vi "Merge Image Manager.vi"(7 "Calling VI Ref":refnum<vi>) -> ()   [LabVIEW 2016]
uses:
  Merge Image Type Defs/Merge Image - Image Control.ctl
  <vilib>/Utility/miscctls.llb/LVPointTypeDef.ctl
  <vilib>/vision/Image Controls.llb/IMAQ Image.ctl
  Merge Image Type Defs/Merge Image - Notifier Type.ctl
  Merge Image Type Defs/Merge Image - Actions.ctl
  <vilib>/vision/NI_Vision_Development_Module.lvlib
panel:
  in  "Blue LUT":cluster{"Blue Min (%)":i32, "Blue Max (%)":i32}={"Blue Min (%)"=0, "Blue Max (%)"=100} {"Blue Max (%)" max=100; "Blue Min (%)" max=100}
  in  "Green LUT":T1={"Green Min (%)"=0, "Green Max (%)"=100} {"Green Max (%)" max=100; "Green Min (%)" max=100}
  in  "Red LUT":cluster{"Red Min (%)":i32, "Red Max (%)":i32}={"Red Min (%)"=0, "Red Max (%)"=100} {"Red Max (%)" max=100; "Red Min (%)" max=100}
  in  "Update Time (ms)":i32=50 min=10 max=300000 step=1
  in  "Load Trans":bool
  in  "Save Trans":bool
  in  "Blue Image":T2 {"Image" items=["None", "Img 01", "Img 02", "Img 03"]}
  in  "Green Image":T2 {"Image" items=["None", "Img 01", "Img 02", "Img 03"]}
  in  "Red Image":T2 {"Image" items=["None", "Img 01", "Img 02", "Img 03"]}
  in  "Image Display":bool
  in  "Quit":bool
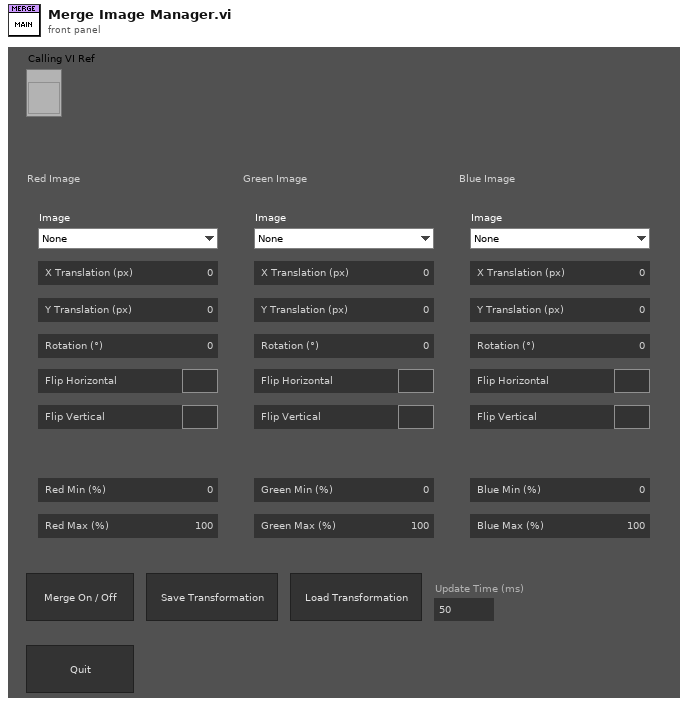
[diagram p1: front panel]
types:
  T1 = cluster{"Green Min (%)":i32, "Green Max (%)":i32}
  T2 = typedef "Merge Image - Image Control.ctl" = cluster{"Image":i32, "X Translation (px)":i32, "Y Translation (px)":i32, "Rotation (°)":sgl, "Flip Horizontal":bool, "Flip Vertical":bool}
  T3 = typedef "Image Type" = u32
  T4 = typedef "Merge Image - Actions.ctl" = enum16{"Timeout", "Update Image Source", "Update LUTs", "Quit"}
  T5 = typedef "Merge Image - Notifier Type.ctl" = cluster{"Actions":T4, "Merge Contols":T2[], "LUT Controls":cluster{"Red Min (%)":i32, "Red Max (%)":i32}[]}
  T6 = typedef "IMAQ Image.ctl" = refnum<image>
  T7 = enum16{"Always On", "Always Off", "Off While Running"}
  T8 = typedef "LVPointTypeDef.ctl" = cluster{"Horizontal":i16, "Vertical":i16}
  T9 = enum32{"Invalid", "Standard", "Closed", "Hidden", "Minimized", "Maximized"}
  T10 = typedef "LVRectTypeDef.ctl" = cluster{"Left":i16, "Top":i16, "Right":i16, "Bottom":i16}
  T11 = typedef "LVBoundsTypeDef.ctl" = cluster{"Width":u32, "Height":u32}
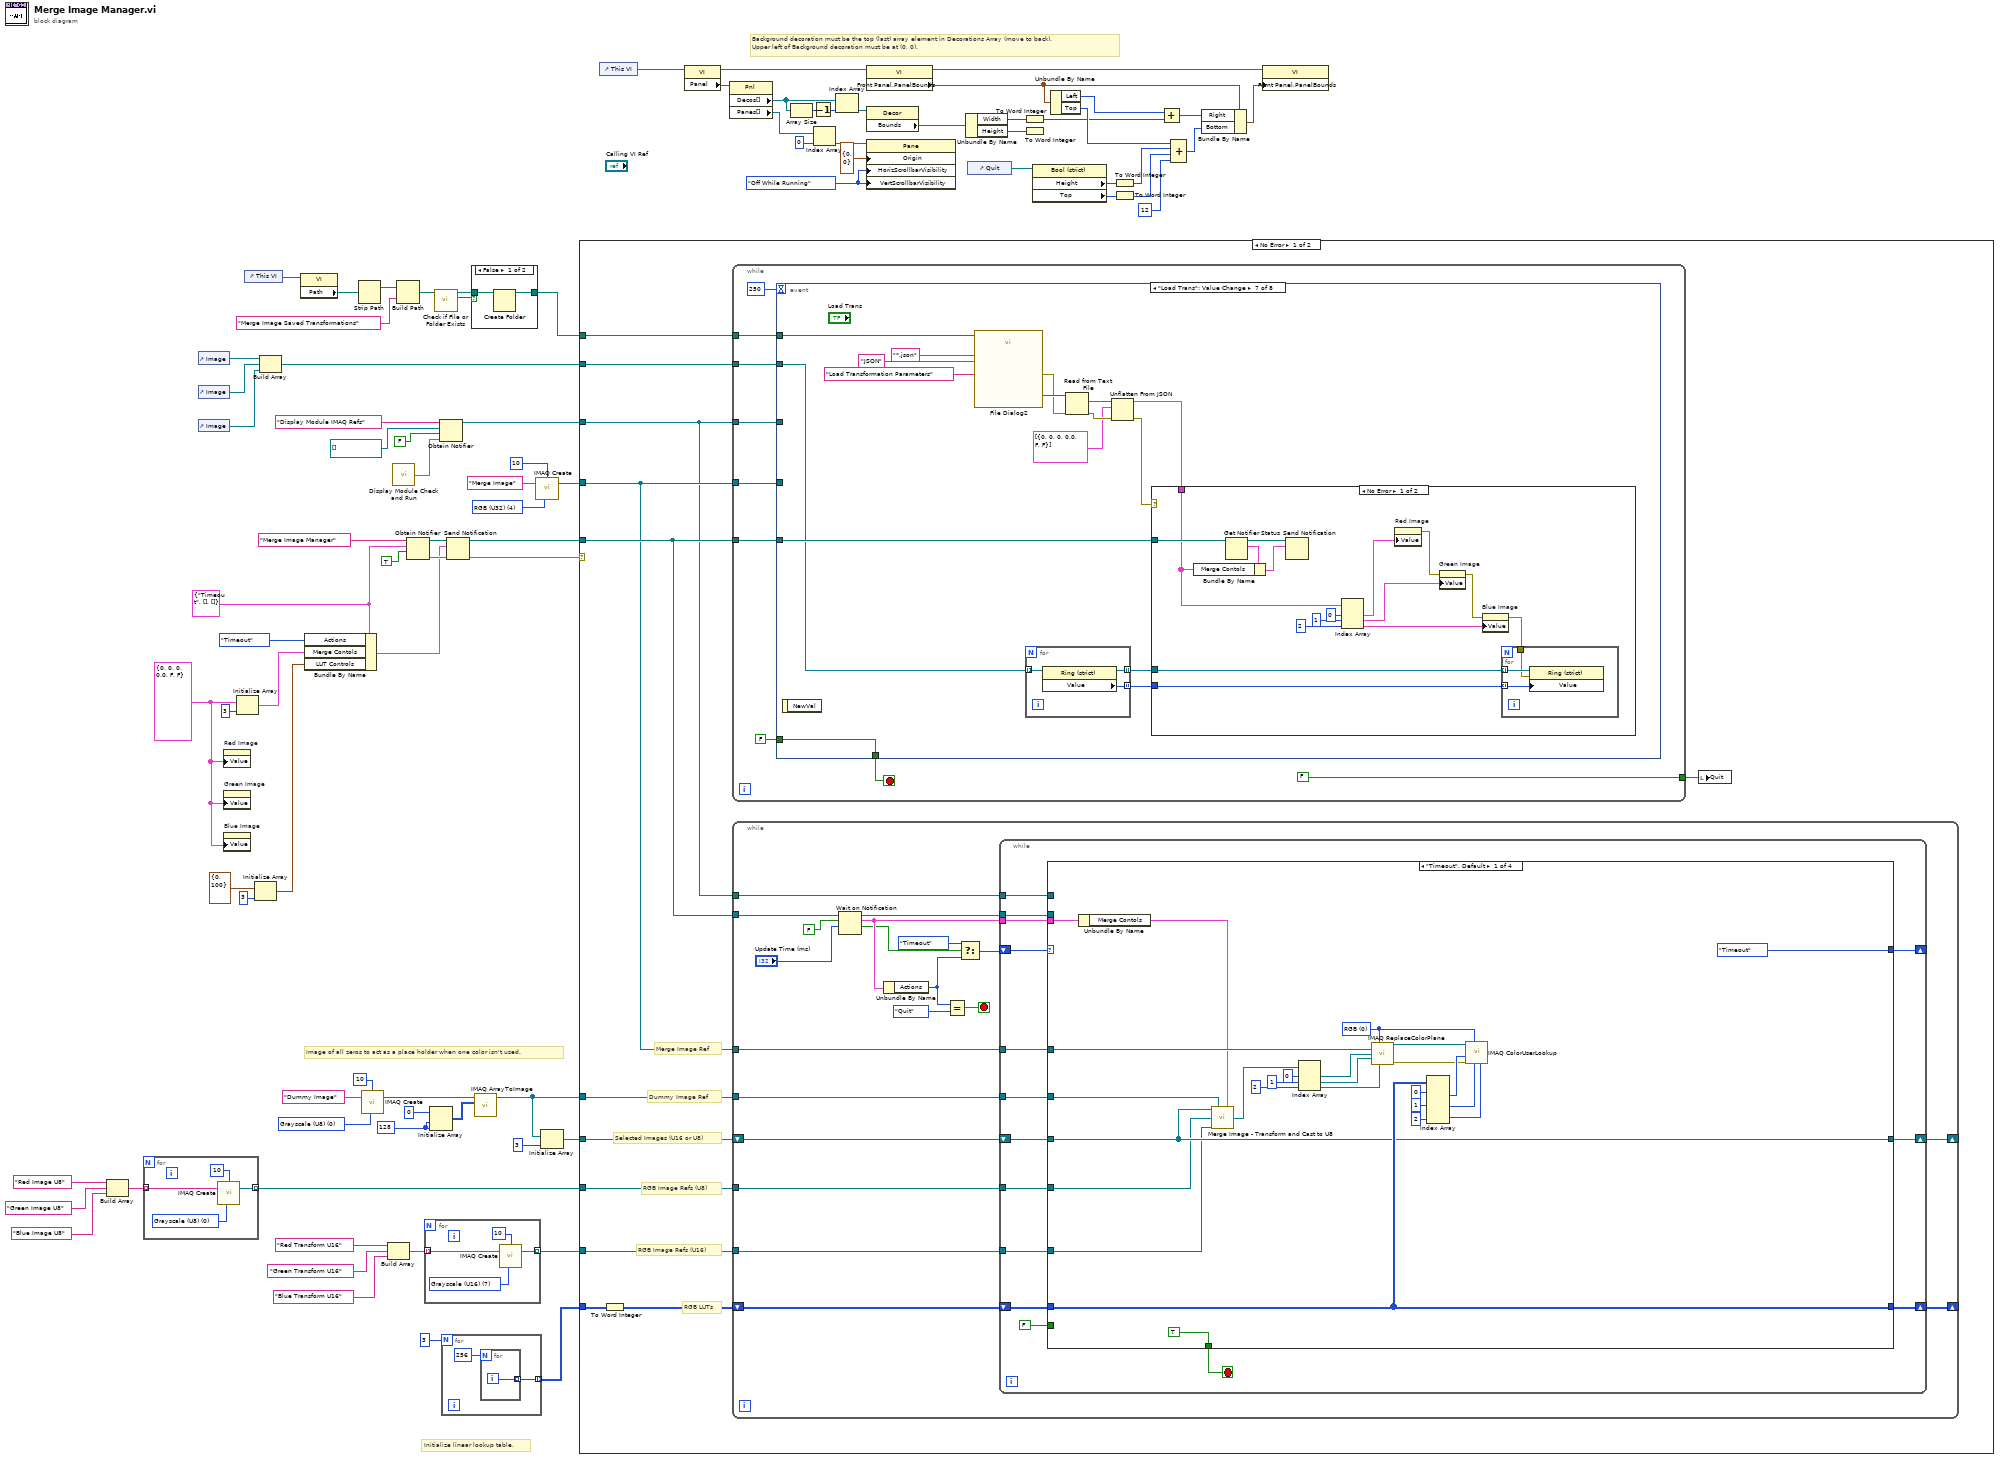
[diagram p0: block diagram]
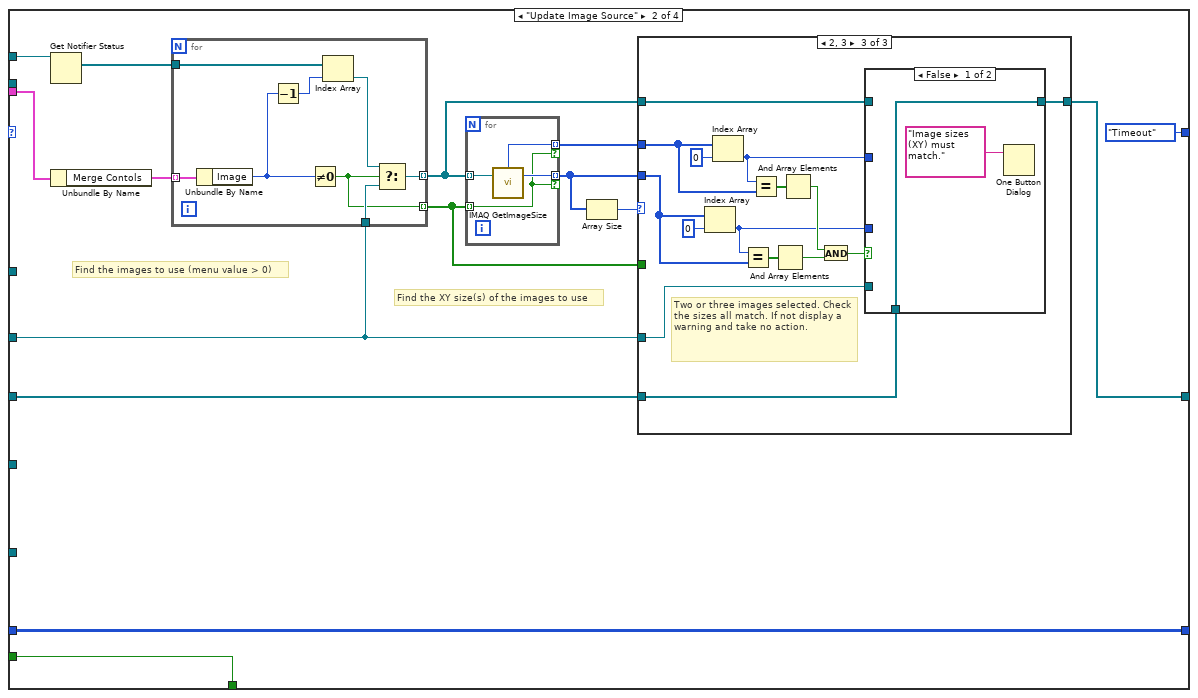
[diagram p3: hidden frame]
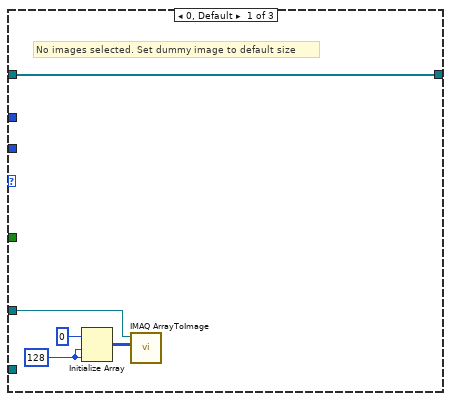
[diagram p4: hidden frame]
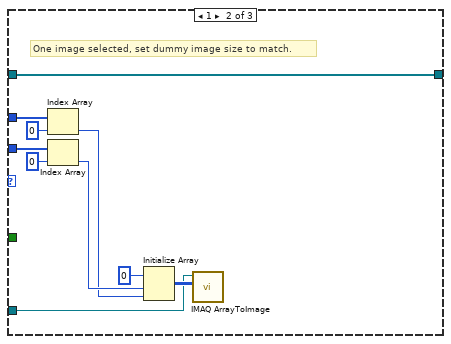
[diagram p5: hidden frame]
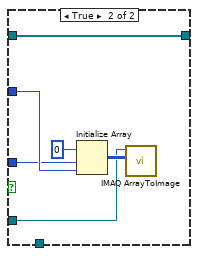
[diagram p6: hidden frame]
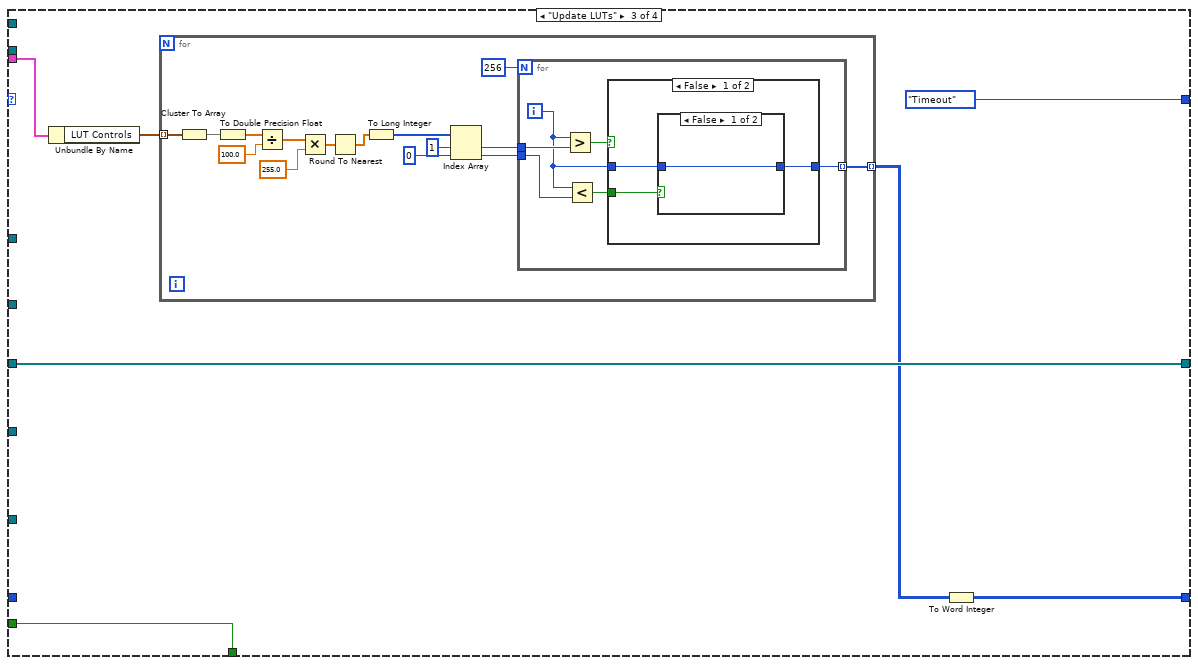
[diagram p7: hidden frame]
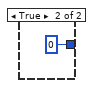
[diagram p8: hidden frame]
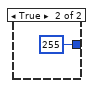
[diagram p9: hidden frame]
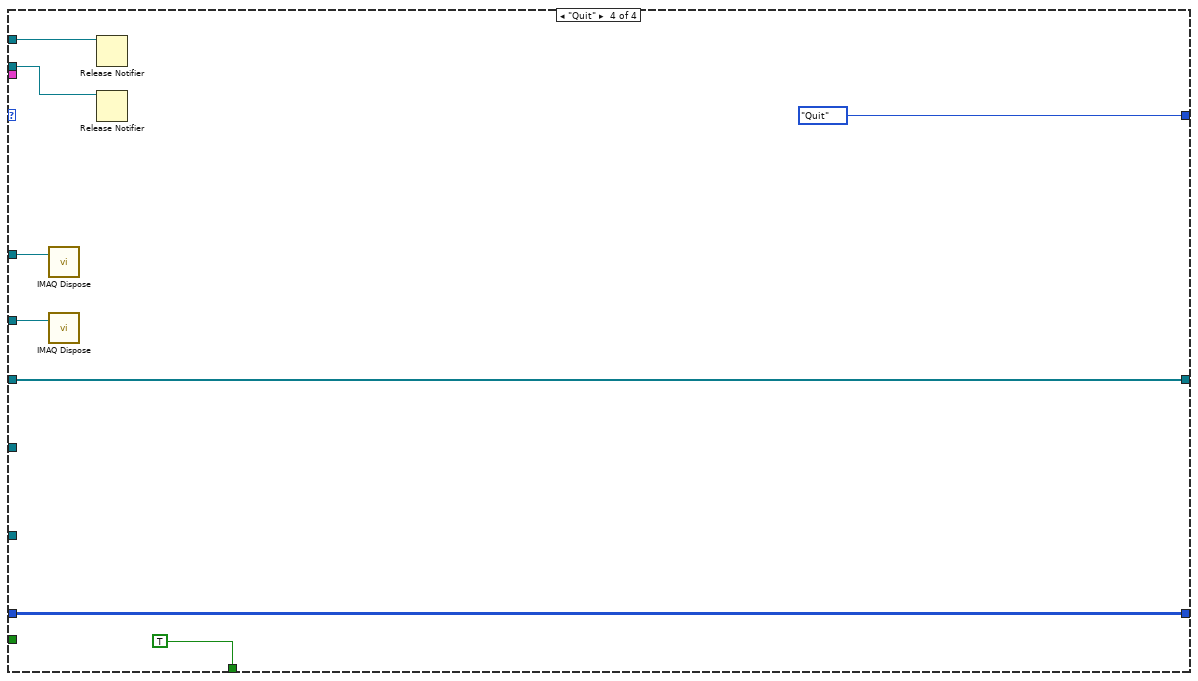
[diagram p10: hidden frame]
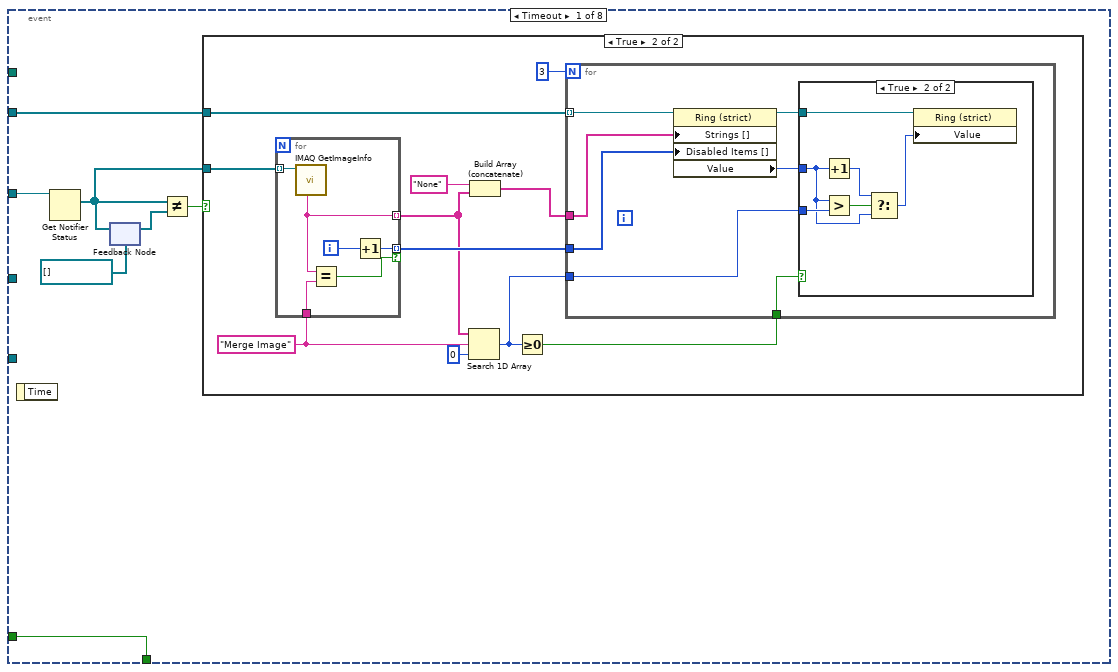
[diagram p11: hidden frame]
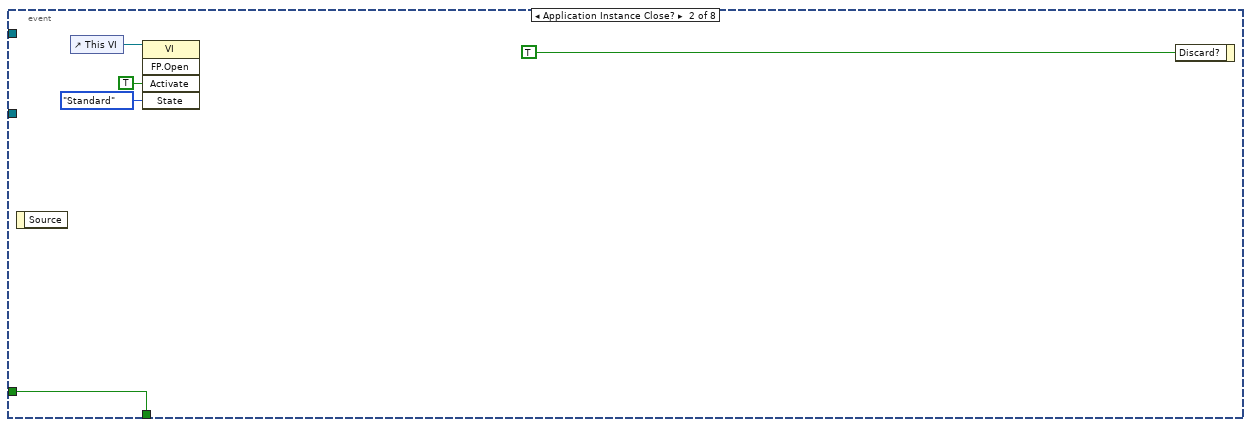
[diagram p14: hidden frame]
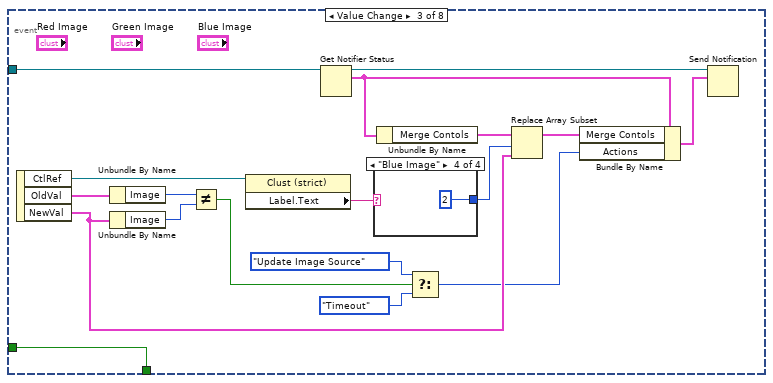
[diagram p15: hidden frame]
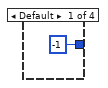
[diagram p16: hidden frame]
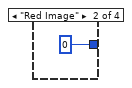
[diagram p17: hidden frame]
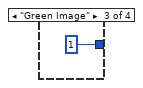
[diagram p18: hidden frame]
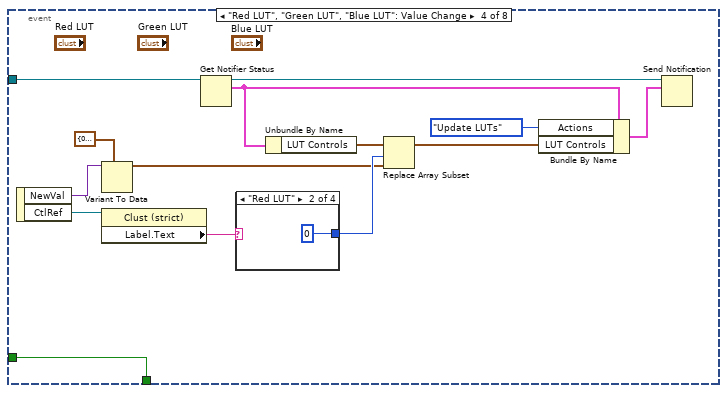
[diagram p19: hidden frame]
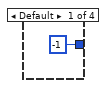
[diagram p20: hidden frame]
diagram:
  w18 = 128 ("dimension size")
  w23 = T3 0 items=["Grayscale (U8)", "Grayscale (I16)", "Grayscale (SGL)", "Complex (CSG)", "RGB (U32)", "HSL (U32)", "RGB (U64)", "Grayscale (U16)"] ("Image Type")
  w2 = T2 {"Image"=0, "X Translation (px)"=0, "Y Translation (px)"=0, "Rotation (°)"=0.0, "Flip Horizontal"=FALSE, "Flip Vertical"=FALSE} ("Image Controls")
  w32 = T5 {"Actions"=enum."Timeout", "Merge Contols"=[], "LUT Controls"=[]} ("Merge Image Notifier Type")
  w41 = T3 4 items=["Grayscale (U8)", "Grayscale (I16)", "Grayscale (SGL)", "Complex (CSG)", "RGB (U32)", "HSL (U32)", "RGB (U64)", "Grayscale (U16)"] ("Image Type")
  w70 = T7."Off While Running" ("Vertical Scrollbar Visibility")
  # "Image of all zeros to act as a place holder when one color isn't used."
  # "Initialize linear lookup table."
  # "Background decoration must be the top (last) array element in Decorations Array (move to back).\nUpper left of Background decoration must be at (0, 0)."
  n1 = Build Array("Red Image U8" ("Image Name"), "Green Image U8" ("Image Name"), "Blue Image U8" ("Image Name")) -> (w12:string[])
  n2 = for {
    tunnel: w12 -> [w89] mode=indexing
    tunnel: [w88] -> w11 mode=indexing
    w90 = T3 0 items=["Grayscale (U8)", "Grayscale (I16)", "Grayscale (SGL)", "Complex (CSG)", "RGB (U32)", "HSL (U32)", "RGB (U64)", "Grayscale (U16)"] ("Image Type")
    n3 = call "IMAQ Create"("Border Size"=10, "Image Name"=w89, "Image Type"=w90) -> ("New Image"=w88:T6)  [unwired: 2 in, 1 out]
  }
  n4 = control-ref of="Image"() -> (w37:refnum<vi>)
  n5 = control-ref of="Image"() -> (w35:refnum<vi>)
  n6 = control-ref of="Image"() -> (w36:refnum<vi>)
  n7 = property on="Red Image" class="Clust (strict)"("Value"=w2) -> ()  [unwired: 2 in, 2 out]
  n8 = property on="Green Image" class="Clust (strict)"("Value"=w2) -> ()  [unwired: 2 in, 2 out]
  n9 = property on="Blue Image" class="Clust (strict)"("Value"=w2) -> ()  [unwired: 2 in, 2 out]
  n10 = Initialize Array(w2, 3 ("dimension size")) -> (w29:T2[])
  n11 = control-ref of="This VI"() -> (w54:refnum<vi>)
  n12 = Initialize Array(cluster{"Red Min (%)":i32, "Red Max (%)":i32} {"Red Min (%)"=0, "Red Max (%)"=100} ("LUT Controls"), 3 ("dimension size")) -> (w26:cluster{"Red Min (%)":i32, "Red Max (%)":i32}[])
  n13 = Build Array(w37, w35, w36) -> (w34:refnum<vi>[])
  n14 = property class="VI"(reference=w54) -> ("Path"=w53:path)  [unwired: 1 in, 2 out]
  n15 = Bundle By Name(cluster=w32, "Actions"=Merge_Image_-_Actions."Timeout", "Merge Contols"=w29, "LUT Controls"=w26) -> (w25:T5)
  n16 = Strip Path(path=w53) -> (stripped path=w52:path)  [unwired: 1 out]
  n17 = call "IMAQ Create"("Border Size"=10, "Image Name"="Dummy Image", "Image Type"=w23) -> ("New Image"=w24:T6)  [unwired: 2 in, 1 out]
  n18 = Build Array("Red Transform U16" ("Image Name"), "Green Transform U16" ("Image Name"), "Blue Transform U16" ("Image Name")) -> (w7:string[])
  n19 = call "Display Module Check and Run.vi"() -> ("Error"=w33:errorcluster)  [unwired: 15 in]
  n20 = Build Path(base path=w52, name or relative path="Merge Image Saved Transformations") -> (appended path=w50:path)
  n21 = Obtain Notifier(name (unnamed)="Merge Image Manager", notification data type=w32, create if not found? (T)=TRUE) -> (notifier out=w56:refnum<notifier>, error out=w47:errorcluster)  [unwired: 1 in, 1 out]
  n22 = for {
    tunnel: w7 -> [w93] mode=indexing
    tunnel: [w92] -> w3 mode=indexing
    w94 = T3 7 items=["Grayscale (U8)", "Grayscale (I16)", "Grayscale (SGL)", "Complex (CSG)", "RGB (U32)", "HSL (U32)", "RGB (U64)", "Grayscale (U16)"] ("Image Type")
    n23 = call "IMAQ Create"("Border Size"=10, "Image Name"=w93, "Image Type"=w94) -> ("New Image"=w92:T6)  [unwired: 2 in, 1 out]
  }
  n24 = Initialize Array(u8 0 ("element"), w18, w18) -> (w19:u8[][])
  n25 = call <vilib>:"Check if File or Folder Exists.vi"("path"=w50) -> ("file or folder exists?"=w49:bool, "dup path"=w48:path)  [unwired: 8 in, 1 out]
  n26 = Obtain Notifier(name (unnamed)="Display Module IMAQ Refs", notification data type=T6[] [], create if not found? (T)=FALSE, error in (no error)=w33) -> (notifier out=w38:refnum<notifier>)  [unwired: 2 out]
  n27 = for {
    N: 3 -> [_]
    tunnel: [w96] -> w16 mode=indexing
    n28 = for {
      N: 256 -> [_]
      tunnel: [w98] -> w96 mode=indexing
      i -> [w98]
    }
  }
  n29 = Send Notification(notification=w25, notifier=w56, error in (no error)=w47) -> (notifier out=w55:refnum<notifier>, error out=w46:errorcluster)
  n30 = case shown="False" w49 {
    tunnel: w48 -> [w100 w101]
    tunnel: [w99 w101] -> w1
    frame False {
      n31 = Create Folder(path (use dialog)=w100) -> (created path=w99:path)  [unwired: 2 in, 2 out]
    }
    frame True {
    }
  }
  n32 = call "IMAQ ArrayToImage"("Image Pixels (U8)"=w19, "Image"=w24) -> ("Image Out"=w8:T6)  [unwired: 8 in, 1 out]
  n33 = call "IMAQ Create"("Border Size"=10, "Image Name"="Merge Image", "Image Type"=w41) -> ("New Image"=w39:T6)  [unwired: 2 in, 1 out]
  n34 = Initialize Array(w8, 3 ("dimension size")) -> (w9:T6[])
  n35 = case shown="No Error" w46 {
    selector: w46 -> [_ w471]
    tunnel: w55 -> [w112 w473]
    tunnel: w39 -> [w108 w472]
    tunnel: w38 -> [w107 w474]
    tunnel: w34 -> [w111 _]
    tunnel: w8 -> [w110 _]
    tunnel: w11 -> [w106 _]
    tunnel: w16 -> [w109 _]
    tunnel: w9 -> [w105 _]
    tunnel: w3 -> [w104 _]
    tunnel: w1 -> [w102 _]
    frame No Error {
      # "RGB Image Refs (U16)"
      # "Selected Images (U16 or U8)"
      # "Merge Image Ref"
      # "Dummy Image Ref"
      # "RGB Image Refs (U8)"
      # "RGB LUTs"
      n36 = To Word Integer(number=w109) -> (16bit integer=w103:i16[][])
      n37 = while {
        tunnel: w112 -> [w288]
        tunnel: [FALSE] -> w113
        tunnel: w108 -> [w286]
        tunnel: w107 -> [w285]
        tunnel: w111 -> [w284]
        tunnel: w102 -> [w282]
        stop <- w289 stop-if-true
        n38 = event shown="[6] \"Load Trans\": Value Change" {
          selector: _ -> [_ _ _ _ _ _ _ _]
          dyn-events: _ -> [_ _ _ _ _ _ _ _]
          timeout: 250 -> [_ _ _ _ _ _ _ _]
          tunnel: FALSE -> [w297 w331 w350 w368 w383 w422 w440 _]
          tunnel: [w297 w331 w350 w368 w383 w422 w440 w468] -> w289
          tunnel: w288 -> [_ _ w349 w367 _ w421 w430 w467]
          tunnel: w286 -> [_ _ _ _ w375 _ _ _]
          tunnel: w285 -> [w296 _ _ _ w374 _ _ _]
          tunnel: w284 -> [w292 _ _ _ w373 _ w427 _]
          tunnel: w282 -> [_ _ _ _ _ w418 w435 _]
          event Timeout {
            n39 = event-data() -> ()  [unwired: 1 in, 1 out]
            n40 = Get Notifier Status(notifier=w296) -> (current notification=w291:T6[])  [unwired: 1 in, 4 out]
            n41 = feedback-in #1(w291) -> ()
            n42 = feedback #1(T6[] []) -> (w294:T6[])
            n43 = Not Equal?(x=w291, y=w294) -> (x != y?=w293:bool)
            n44 = case shown="True" w293 {
              tunnel: w292 -> [_ w307]
              tunnel: w291 -> [_ w308]
              frame False {
              }
              frame True {
                w301 = "Merge Image" ("Image Name")
                n45 = for {
                  tunnel: w308 -> [w327] mode=indexing
                  tunnel: [w326] -> w302 mode=indexing
                  tunnel: [w325] -> w303 mode=indexing if=w323
                  tunnel: w301 -> [w322]
                  i -> [w324]
                  n46 = call "IMAQ GetImageInfo"("Image"=w327) -> ("Image Name"=w326:string)  [unwired: 3 in, 7 out]
                  n47 = Equal?(x=w326, y=w322) -> (x = y?=w323:bool)
                  n48 = Increment(x=w324) -> (x+1=w325:i32)
                }
                n49 = Search 1D Array(1D array=w302, element=w301, start index (0)=0) -> (index of element=w298:i32)
                n50 = Build Array (concatenate)("None", w302) -> (w305:string[])
                n51 = Greater Or Equal To 0?(x=w298) -> (x >= 0?=w299:bool)
                n52 = for {
                  N: 3 -> [_]
                  tunnel: w307 -> [w315] mode=indexing
                  tunnel: w305 -> [w314]
                  tunnel: w303 -> [w313]
                  tunnel: w299 -> [w310]
                  tunnel: w298 -> [w309]
                  n53 = property class="Ring (strict)"(reference=w315, "Strings []"=w314, "Disabled Items []"=w313) -> (reference out=w312:refnum<vi>, "Value"=w311:i32)  [unwired: 1 in, 1 out]
                  n54 = case shown="True" w310 {
                    tunnel: w312 -> [_ w321]
                    tunnel: w311 -> [_ w316]
                    tunnel: w309 -> [_ w320]
                    frame False {
                    }
                    frame True {
                      n55 = Increment(x=w316) -> (x+1=w318:i32)
                      n56 = Greater?(x=w316, y=w320) -> (0:w319:bool)
                      n57 = Select(t=w318, s=w319, f=w316) -> (s? t:f=w317:i32)
                      n58 = property class="Ring (strict)"(reference=w321, "Value"=w317) -> ()  [unwired: 1 in, 2 out]
                    }
                  }
                }
              }
            }
          }
          event Application Instance Close? {
            n59 = event-data() -> ()  [unwired: 1 in, 1 out]
            n60 = control-ref of="This VI"() -> (w328:refnum<vi>)
            n61 = invoke class="VI" method="FP.Open"(reference=w328, "Activate"=TRUE ("Activate?"), "State"=T9."Standard") -> ()  [unwired: 2 in, 5 out]
            n62 = event-data("Discard?"=TRUE) -> ()  [unwired: 1 in, 1 out]
          }
          event Value Change {
            n63 = event-data() -> ("CtlRef"=w347:refnum<vi>, "OldVal"=w340:T2, "NewVal"=w337:T2)  [unwired: 1 in]
            n64 = Unbundle By Name(w340) -> ("Image"=w339:i32)
            n65 = Unbundle By Name(w337) -> ("Image"=w338:i32)
            n66 = Not Equal?(x=w339, y=w338) -> (x != y?=w336:bool)
            n67 = property class="Clust (strict)"(reference=w347) -> ("Label.Text"=w346:string)  [unwired: 1 in, 2 out]
            n68 = Get Notifier Status(notifier=w349) -> (notifier out=w348:refnum<notifier>, current notification=w341:T5)  [unwired: 1 in, 3 out]
            n69 = case shown="\"Blue Image\"" w346 {
              tunnel: [-1 0 1 2] -> w344
              frame Default {
              }
              frame "Red Image" {
              }
              frame "Green Image" {
              }
              frame "Blue Image" {
              }
            }
            n70 = Unbundle By Name(w341) -> ("Merge Contols"=w345:T2[])
            n71 = Select(t=Merge_Image_-_Actions."Update Image Source" ("Actions"), s=w336, f=Merge_Image_-_Actions."Timeout" ("Actions")) -> (s? t:f=w333:T4)
            n72 = Replace Array Subset(array=w345, new element=w337, index=w344) -> (w343:T2[])
            n73 = Bundle By Name(cluster=w341, "Merge Contols"=w343, "Actions"=w333) -> (w342:T5)
            n74 = Send Notification(notification=w342, notifier=w348) -> ()  [unwired: 1 in, 2 out]
          }
          event "Red LUT", "Green LUT", "Blue LUT": Value Change {
            n75 = event-data() -> ("NewVal"=w357:variant, "CtlRef"=w358:refnum<vi>)  [unwired: 1 in]
            n76 = Variant To Data(type=cluster{"Red Min (%)":u16, "Red Max (%)":u16} {"Red Min (%)"=0, "Red Max (%)"=100} ("LUT Controls"), Variant=w357) -> (data=w355:cluster{"Red Min (%)":u16, "Red Max (%)":u16})  [unwired: 1 in, 1 out]
            n77 = property class="Clust (strict)"(reference=w358) -> ("Label.Text"=w365:string)  [unwired: 1 in, 2 out]
            n78 = Get Notifier Status(notifier=w367) -> (notifier out=w366:refnum<notifier>, current notification=w359:T5)  [unwired: 1 in, 3 out]
            n79 = case shown="\"Red LUT\"" w365 {
              tunnel: [-1 0 1 2] -> w363
              frame Default {
              }
              frame "Red LUT" {
              }
              frame "Green LUT" {
              }
              frame "Blue LUT" {
              }
            }
            n80 = Unbundle By Name(w359) -> ("LUT Controls"=w364:cluster{"Red Min (%)":i32, "Red Max (%)":i32}[])
            n81 = Replace Array Subset(array=w364, new element=w355, index=w363) -> (w362:cluster{"Red Min (%)":i32, "Red Max (%)":i32}[])
            n82 = Bundle By Name(cluster=w359, "Actions"=Merge_Image_-_Actions."Update LUTs", "LUT Controls"=w362) -> (w360:T5)
            n83 = Send Notification(notification=w360, notifier=w366) -> ()  [unwired: 1 in, 2 out]
          }
          event "Image Display": Value Change {
            n84 = event-data() -> ("NewVal"=w376:bool)  [unwired: 1 in]
            n85 = Get Notifier Status(notifier=w374) -> (notifier out=w382:refnum<notifier>, current notification=w380:T6[], error out=w381:errorcluster)  [unwired: 1 in, 2 out]
            n86 = case shown="False" w376 {
              tunnel: w382 -> [w392 w409]
              tunnel: w381 -> [w390 w408]
              tunnel: w380 -> [w389 w407]
              tunnel: [w391 w405] -> w377
              tunnel: [w392 w409] -> w379
              tunnel: [w390 w408] -> w378
              tunnel: w375 -> [w388 w406]
              tunnel: w373 -> [w385 _]
              frame False {
                n87 = Search 1D Array(1D array=w389, element=w388, start index (0)=0) -> (index of element=w384:i32)
                n88 = Greater Or Equal To 0?(x=w384) -> (x >= 0?=w386:bool)
                n89 = case shown="True" w386 {
                  tunnel: w384 -> [_ w403]
                  tunnel: w389 -> [w400 w402]
                  tunnel: [w400 w401] -> w391
                  frame False {
                  }
                  frame True {
                    n90 = Delete From Array(array=w402, length=1, index=w403) -> (array with subset deleted=w401:T6[])  [unwired: 1 out]
                  }
                }
                n91 = for {
                  tunnel: w385 -> [w399] mode=indexing
                  tunnel: w384 -> [w397]
                  n92 = property class="Ring (strict)"(reference=w399) -> (reference out=w398:refnum<vi>, "Value"=w393:i32)  [unwired: 1 in, 1 out]
                  n93 = Greater?(x=w393, y=w397) -> (0:w396:bool)
                  n94 = Decrement(x=w393) -> (x-1=w395:i32)
                  n95 = Select(t=w395, s=w396, f=w393) -> (s? t:f=w394:i32)
                  n96 = property class="Ring (strict)"(reference=w398, "Value"=w394) -> ()  [unwired: 1 in, 2 out]
                }
              }
              frame True {
                n97 = Build Array (concatenate)(w407, w406) -> (w405:T6[])
              }
            }
            n98 = Send Notification(notification=w377, notifier=w379, error in (no error)=w378) -> ()  [unwired: 2 out]
          }
          event "Save Trans": Value Change {
            n99 = event-data() -> ()  [unwired: 1 in, 1 out]
            n100 = Get Notifier Status(notifier=w421) -> (current notification=w420:T5, error out=w411:errorcluster)  [unwired: 1 in, 3 out]
            n101 = Unbundle By Name(w420) -> ("Merge Contols"=w419:T2[])
            n102 = Flatten To JSON(anything=w419, error in (no error)=w411) -> (JSON string=w412:string, 11:w410:errorcluster)  [unwired: 1 in]
            n103 = call "File Dialog"("start path"=w418, "prompt"="Save Transformation Parameters", "error in"=w410, "pattern (all files)"="*.json", "pattern label"="JSON") -> ("selected path"=w413:path, "error out"=w414:errorcluster)  [unwired: 7 in, 2 out]
            n104 = case shown="No Error" w414 {
              tunnel: w413 -> [w424 _]
              tunnel: w412 -> [w423 _]
              frame No Error {
                n105 = Write to Text File(file (use dialog)=w424, text=w423) -> ()  [unwired: 2 in, 3 out]
              }
              frame Error {
              }
            }
          }
          event "Load Trans": Value Change {
            n106 = event-data() -> ()  [unwired: 1 in, 1 out]
            n107 = call "File Dialog2"("start path"=w435, "prompt"="Load Transformation Parameters", "pattern (all files)"="*.json", "pattern label"="JSON") -> ("selected path"=w436:path, "error out"=w434:errorcluster)  [unwired: 8 in, 2 out]
            n108 = for {
              tunnel: w427 -> [w443] mode=indexing
              tunnel: [w442] -> w425 mode=indexing
              tunnel: [w441] -> w426 mode=indexing
              n109 = property class="Ring (strict)"(reference=w443) -> (reference out=w441:refnum<vi>, "Value"=w442:i32)  [unwired: 1 in, 1 out]
            }
            n110 = Read from Text File(file (use dialog)=w436, error in=w434) -> (text=w433:string, error out=w432:errorcluster)  [unwired: 2 in, 2 out]
            n111 = Unflatten From JSON(JSON string=w433, type and defaults=T2[] [{"Image"=0, "X Translation (px)"=0, "Y Translation (px)"=0, "Rotation (°)"=0.0, "Flip Horizontal"=FALSE, "Flip Vertical"=FALSE}], error in (no error)=w432) -> (value=w429:T2[], error out=w428:errorcluster)  [unwired: 4 in]
            n112 = case shown="No Error" w428 {
              tunnel: w430 -> [w459 _]
              tunnel: w429 -> [w455 _]
              tunnel: w426 -> [w448 _]
              tunnel: w425 -> [w447 _]
              frame No Error {
                n113 = Get Notifier Status(notifier=w459) -> (notifier out=w458:refnum<notifier>, current notification=w457:T5)  [unwired: 1 in, 3 out]
                n114 = Bundle By Name(cluster=w457, "Merge Contols"=w455) -> (w456:T5)
                n115 = Send Notification(notification=w456, notifier=w458) -> ()  [unwired: 1 in, 2 out]
                n116 = Index Array(array=w455, index #1=0 ("index"), index #2=1 ("index"), index #3=2 ("index")) -> (element #1=w451:T2, element #2=w450:T2, element #3=w449:T2)
                n117 = property on="Red Image" class="Clust (strict)"("Value"=w451) -> (error out=w446:errorcluster)  [unwired: 2 in, 1 out]
                n118 = property on="Green Image" class="Clust (strict)"(error in=w446, "Value"=w450) -> (error out=w445:errorcluster)  [unwired: 1 in, 1 out]
                n119 = property on="Blue Image" class="Clust (strict)"(error in=w445, "Value"=w449) -> (error out=w444:errorcluster)  [unwired: 1 in, 1 out]
                n120 = for {
                  tunnel: w448 -> [w462] mode=indexing
                  tunnel: w447 -> [w461] mode=indexing
                  tunnel: w444 -> [w460]
                  n121 = property class="Ring (strict)"(reference=w462, error in=w460, "Value"=w461) -> ()  [unwired: 2 out]
                }
              }
              frame Error {
              }
            }
          }
          event "Quit": Value Change {
            n122 = event-data() -> ("NewVal"=w468:bool)  [unwired: 1 in]
            n123 = Get Notifier Status(notifier=w467) -> (notifier out=w466:refnum<notifier>, current notification=w465:T5)  [unwired: 1 in, 3 out]
            n124 = Bundle By Name(cluster=w465, "Actions"=Merge_Image_-_Actions."Quit") -> (w463:T5)
            n125 = Send Notification(notification=w463, notifier=w466) -> ()  [unwired: 1 in, 2 out]
          }
        }
      }
      n126 = while {
        tunnel: w112 -> [w133]
        tunnel: w110 -> [w122]
        shift-right: [w119] -> _
        shift-left: w105 -> [w121]
        shift-right: [w118] -> _
        shift-left: w103 -> [w120]
        tunnel: w108 -> [w117]
        tunnel: w107 -> [w116]
        tunnel: w106 -> [w115]
        tunnel: w104 -> [w114]
        stop <- w131 stop-if-true
        n127 = Wait on Notification(notifier=w133, ignore previous (F)=FALSE, timeout in ms (-1)="Update Time (ms)") -> (notifier out=w129:refnum<notifier>, notification=w130:T5, timed out?=w127:bool)  [unwired: 1 in, 1 out]
        n128 = Unbundle By Name(w130) -> ("Actions"=w126:T4)
        n129 = Equal?(x=w126, y=Merge_Image_-_Actions."Quit") -> (x = y?=w131:bool)
        n130 = Select(t=Merge_Image_-_Actions."Timeout", s=w127, f=w126) -> (s? t:f=w124:T4)
        n131 = while {
          shift-right: [w146] -> _
          shift-left: w124 -> [w148]
          tunnel: w130 -> [w147]
          tunnel: w129 -> [w145]
          tunnel: w122 -> [w142]
          tunnel: w117 -> [w136]
          tunnel: w116 -> [w137]
          shift-right: [w139] -> w119
          shift-left: w121 -> [w141]
          tunnel: w115 -> [w135]
          tunnel: w114 -> [w134]
          shift-right: [w138] -> w118
          shift-left: w120 -> [w140]
          stop <- w143 stop-if-true
          n132 = case shown="\"Timeout\", Default" w148 {
            tunnel: w147 -> [w168 w186 w243 _]
            tunnel: [Merge_Image_-_Actions."Timeout" ("y") Merge_Image_-_Actions."Timeout" ("y") Merge_Image_-_Actions."Timeout" ("y") Merge_Image_-_Actions."Quit" ("y")] -> w146
            tunnel: w145 -> [_ _ _ w275]
            tunnel: FALSE -> [_ w189 w245 _]
            tunnel: [TRUE w189 w245 TRUE] -> w143
            tunnel: w142 -> [w167 w175 _ w279]
            tunnel: w141 -> [w171 w176 w244 w277]
            tunnel: w140 -> [w172 w187 _ w278]
            tunnel: [w171 w177 w244 w277] -> w139
            tunnel: [w172 w187 w240 w278] -> w138
            tunnel: w137 -> [_ w184 _ w274]
            tunnel: w136 -> [w173 _ _ w276]
            tunnel: w135 -> [w170 _ _ _]
            tunnel: w134 -> [w169 _ _ _]
            frame "Timeout", Default {
              w157 = u16 0 items=["RGB", "HSL", "HSV", "HSI"] ("Color Mode")
              n133 = Unbundle By Name(w168) -> ("Merge Contols"=w166:T2[])
              n134 = call "Merge Image - Transform and Cast to U8.vi"("Selected Image (U8 or U16)"=w171, "Dummy Image Ref"=w167, "Transform Parameters"=w166, "RGB Image Refs (U8)"=w170, "RGB Image Refs (U16)"=w169) -> ("RGB Image Refs (U8 DUP)"=w165:T6[])  [unwired: 10 in]
              n135 = Index Array(array=w165, index #1=0 ("index"), index #2=1 ("index"), index #3=2 ("index")) -> (element #1=w161:T6, element #2=w160:T6, element #3=w159:T6)
              n136 = call "IMAQ ReplaceColorPlane"("Color Mode"=w157, "Image Dst"=w173, "Red or Hue Plane"=w161, "Green or Sat Plane"=w160, "Blue or Luma or Val or Inten Plane"=w159) -> ("Image Dst Out"=w150:T6, "error out"=w149:errorcluster)  [unwired: 9 in]
              n137 = Index Array(array=w172, index (row) #1=0 ("index (row)"), index (row) #2=1 ("index (row)"), index (row) #3=2 ("index (row)")) -> (element #1=w153:i16[], element #2=w152:i16[], element #3=w151:i16[])  [unwired: 3 in]
              n138 = call "IMAQ ColorUserLookup"("Blue or Luma or Val or Inten Lookup Table"=w151, "Green or Sat Lookup Table"=w152, "Color Mode"=w157, "error in (no error)"=w149, "Red or Hue Lookup Table"=w153, "Image Src"=w150) -> ()  [unwired: 4 in, 2 out]
            }
            frame "Update Image Source" {
              # "Find the XY size(s) of the images to use"
              # "Find the images to use (menu value > 0)"
              n139 = Get Notifier Status(notifier=w184) -> (current notification=w183:T6[])  [unwired: 1 in, 4 out]
              n140 = Unbundle By Name(w186) -> ("Merge Contols"=w185:T2[])
              n141 = for {
                tunnel: w185 -> [w239] mode=indexing
                tunnel: w183 -> [w238]
                tunnel: [w234] -> w178 mode=indexing
                tunnel: w175 -> [w233]
                tunnel: [w232] -> w179 mode=indexing
                n142 = Unbundle By Name(w239) -> ("Image"=w237:i32)
                n143 = Decrement(x=w237) -> (x-1=w236:i32)
                n144 = Not Equal To 0?(x=w237) -> (x != 0?=w232:bool)
                n145 = Index Array(array=w238, index=w236) -> (element=w235:T6)
                n146 = Select(t=w235, s=w232, f=w233) -> (s? t:f=w234:T6)
              }
              n147 = for {
                tunnel: w178 -> [w231] mode=indexing
                tunnel: w179 -> [w228] mode=indexing
                tunnel: [w230] -> w181 mode=indexing if=w228
                tunnel: [w229] -> w180 mode=indexing if=w228
                n148 = call "IMAQ GetImageSize"("Image"=w231) -> ("Y Resolution"=w229:i32, "X Resolution"=w230:i32)  [unwired: 3 in, 1 out]
              }
              n149 = Array Size(array=w180) -> (size(s)=w182:i32)
              n150 = case shown="2, 3" w182 {
                tunnel: w181 -> [_ w204 w214]
                tunnel: w180 -> [_ w201 w217]
                tunnel: w179 -> [_ _ _]
                tunnel: w178 -> [w191 w196 w208]
                tunnel: [w191 w196 w207] -> w177
                tunnel: w176 -> [_ _ w206]
                tunnel: w175 -> [w190 w195 w205]
                frame 0, Default {
                  w193 = 128 ("dimension size")
                  # "No images selected. Set dummy image to default size"
                  n151 = Initialize Array(u8 0 ("element"), w193, w193) -> (w192:u8[][])
                  n152 = call "IMAQ ArrayToImage"("Image Pixels (U8)"=w192, "Image"=w190) -> ()  [unwired: 8 in, 2 out]
                }
                frame 1 {
                  # "One image selected, set dummy image size to match."
                  n153 = Index Array(array=w204, index=0) -> (element=w197:i32)
                  n154 = Index Array(array=w201, index=0) -> (element=w198:i32)
                  n155 = Initialize Array(u8 0 ("element"), w198, w197) -> (w199:u8[][])
                  n156 = call "IMAQ ArrayToImage"("Image Pixels (U8)"=w199, "Image"=w195) -> ()  [unwired: 8 in, 2 out]
                }
                frame 2, 3 {
                  # "Two or three images selected. Check the sizes all match. If not display a warning and take no action."
                  n157 = Index Array(array=w217, index=0) -> (element=w209:i32)
                  n158 = Index Array(array=w214, index=0) -> (element=w210:i32)
                  n159 = Equal?(x=w209, y=w217) -> (x = y?=w216:bool[])
                  n160 = Equal?(x=w210, y=w214) -> (x = y?=w215:bool[])
                  n161 = And Array Elements(Boolean array=w216) -> (logical AND=w212:bool)
                  n162 = And Array Elements(Boolean array=w215) -> (logical AND=w213:bool)
                  n163 = And(x=w213, y=w212) -> (x .and. y?=w211:bool)
                  n164 = case shown="False" w211 {
                    tunnel: w210 -> [_ w224]
                    tunnel: w209 -> [_ w223]
                    tunnel: w208 -> [_ w227]
                    tunnel: [w221 w227] -> w207
                    tunnel: w205 -> [_ w222]
                    tunnel: w206 -> [w221 _]
                    frame False {
                      n165 = One Button Dialog(message="Image sizes (XY) must match.") -> ()  [unwired: 1 in, 1 out]
                    }
                    frame True {
                      n166 = Initialize Array(u8 0 ("element"), w223, w224) -> (w225:u8[][])
                      n167 = call "IMAQ ArrayToImage"("Image Pixels (U8)"=w225, "Image"=w222) -> ()  [unwired: 8 in, 2 out]
                    }
                  }
                }
              }
            }
            frame "Update LUTs" {
              n168 = Unbundle By Name(w243) -> ("LUT Controls"=w242:cluster{"Red Min (%)":i32, "Red Max (%)":i32}[])
              n169 = for {
                tunnel: w242 -> [w261] mode=indexing
                tunnel: [w257] -> w241 mode=indexing
                n170 = Cluster To Array(cluster=w261) -> (array=w256:i32[])
                n171 = To Double Precision Float(number=w256) -> (double precision float=w255:dbl[])
                n172 = Divide(x=w255, y=100.0) -> (x/y=w253:dbl[])
                n173 = Multiply(x=w253, y=255.0) -> (x*y=w251:dbl[])
                n174 = Round To Nearest(number=w251) -> (nearest integer value=w249:dbl[])
                n175 = To Long Integer(number=w249) -> (32bit integer=w250:i32[])
                n176 = Index Array(array=w250, index #1=1 ("index"), index #2=0 ("index")) -> (element #1=w248:i32, element #2=w247:i32)
                n177 = for {
                  N: 256 -> [_]
                  tunnel: w248 -> [w267]
                  tunnel: w247 -> [w265]
                  tunnel: [w262] -> w257 mode=indexing
                  i -> [w263]
                  n178 = Greater?(x=w263, y=w267) -> (0:w266:bool)
                  n179 = Less?(x=w263, y=w265) -> (x < y?=w264:bool)
                  n180 = case shown="False" w266 {
                    tunnel: w264 -> [w270 _]
                    tunnel: w263 -> [w269 _]
                    tunnel: [w268 255] -> w262
                    frame False {
                      n181 = case shown="False" w270 {
                        tunnel: w269 -> [w271 _]
                        tunnel: [w271 0] -> w268
                        frame False {
                        }
                        frame True {
                        }
                      }
                    }
                    frame True {
                    }
                  }
                }
              }
              n182 = To Word Integer(number=w241) -> (16bit integer=w240:i16[][])
            }
            frame "Quit" {
              n183 = call "IMAQ Dispose"("Image"=w276) -> ()  [unwired: 5 in, 1 out]
              n184 = call "IMAQ Dispose"("Image"=w279) -> ()  [unwired: 5 in, 1 out]
              n185 = Release Notifier(notifier=w274) -> ()  [unwired: 2 in, 3 out]
              n186 = Release Notifier(notifier=w275) -> ()  [unwired: 2 in, 3 out]
            }
          }
        }
      }
      n187 = local write "Quit"(w113) -> ()
    }
    frame Error {
      n188 = Release Notifier(notifier=w473, error in (no error)=w471) -> (error out=w470:errorcluster)  [unwired: 1 in, 2 out]
      n189 = call "IMAQ Dispose"("Image"=w472, "error in (no error)"=w470) -> ("error out"=w469:errorcluster)  [unwired: 4 in]
      n190 = Release Notifier(notifier=w474, error in (no error)=w469) -> ()  [unwired: 1 in, 3 out]
    }
  }
  n191 = control-ref of="This VI"() -> (w62:refnum<vi>)
  n192 = property class="VI"(reference=w62) -> (reference out=w71:refnum<vi>, "Panel"=w63:refnum<vi>)  [unwired: 1 in, 1 out]
  n193 = property class="Pnl"(reference=w63) -> ("Decos[]"=w61:refnum<vi>[], "Panes[]"=w67:refnum<vi>[])  [unwired: 1 in, 2 out]
  n194 = Array Size(array=w61) -> (size(s)=w59:i32)
  n195 = Decrement(x=w59) -> (x-1=w60:i32)
  n196 = Index Array(array=w67, index=0) -> (element=w66:refnum<vi>)
  n197 = Index Array(array=w61, index=w60) -> (element=w69:refnum<vi>)
  n198 = property class="VI"(reference=w71) -> (reference out=w73:refnum<vi>, "Front Panel.PanelBounds"=w74:T10)  [unwired: 1 in, 1 out]
  n199 = property class="Decor"(reference=w69) -> ("Bounds"=w72:T11)  [unwired: 1 in, 2 out]
  n200 = property class="Pane"(reference=w66, "Origin"=T8 {"Horizontal"=0, "Vertical"=0}, "HorizScrollbarVisibility"=w70, "VertScrollbarVisibility"=w70) -> ()  [unwired: 1 in, 2 out]
  n201 = Unbundle By Name(w72) -> ("Width"=w77:u32, "Height"=w80:u32)
  n202 = control-ref of="Quit"() -> (w64:refnum<vi>)
  n203 = To Word Integer(number=w77) -> (16bit integer=w79:i16)
  n204 = To Word Integer(number=w80) -> ()  [unwired: 1 out]
  n205 = property class="Bool (strict)"(reference=w64) -> ("Height"=w82:u32, "Top"=w83:i32)  [unwired: 1 in, 2 out]
  n206 = Unbundle By Name(w74) -> ("Left"=w76:i16, "Top"=w87:i16)
  n207 = To Word Integer(number=w82) -> (16bit integer=w85:i16)
  n208 = To Word Integer(number=w83) -> (16bit integer=w86:i16)
  n209 = Add(x=w76, y=w79) -> (x+y=w78:i16)
  n210 = Compound Arithmetic op=ADD(w87, w85, w86, i16 12 ("y")) -> (w81:i16)
  n211 = Bundle By Name(cluster=w74, "Right"=w78, "Bottom"=w81) -> (w75:T10)
  n212 = property class="VI"(reference=w73, "Front Panel.PanelBounds"=w75) -> ()  [unwired: 1 in, 2 out]
